vi "Send Callback Message.vi"(8 "error in (no error)":errorcluster, 11 "Order Item in":refnum<class "Order Item.lvclass">) -> (0 "error out":errorcluster, 3 "Order Item out":refnum<class "Order Item.lvclass">)   [LabVIEW 2023, in "Order Item.lvclass"]
doc: "Send the callback message provided by the caller. This enables a zero-coupling relationship between the caller and the callee."
uses:
  Order Item.lvclass
  Order Item.lvclass/Order Item.ctl
  <vilib>/ActorFramework/Self-Addressed Msg/Self-Addressed Msg.lvclass
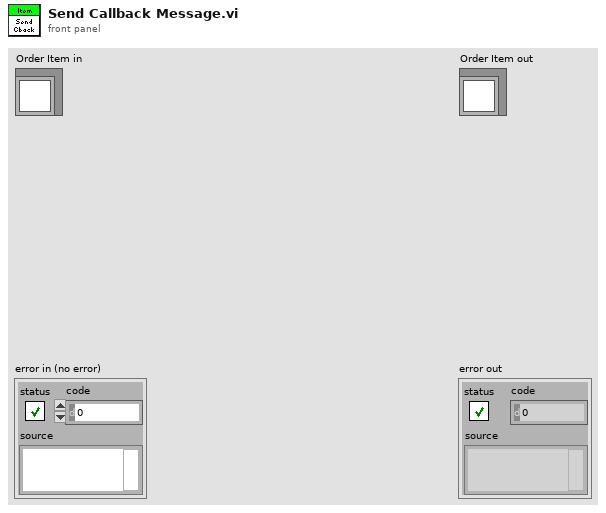
[diagram p1: front panel]
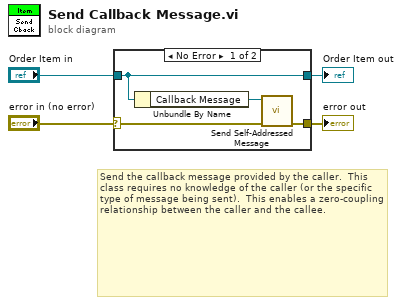
[diagram p0: block diagram]
diagram:
  # "Send the callback message provided by the caller.  This class requires no knowledge of the caller (or the specific type of message being sent).  This enables a zero-coupling relationship between the caller and the callee."
  n1 = case shown="No Error" "error in (no error)" {
    selector: "error in (no error)" -> [w6 w10]
    tunnel: [w5 w10] -> w3
    tunnel: [w8 w9] -> w1
    tunnel: "Order Item in" -> [w8 w9]
    frame No Error {
      n2 = Unbundle By Name(w8) -> ("Callback Message"=w7:refnum<class "Self-Addressed Msg.lvclass">)
      n3 = call-dynamic "Send Self-Addressed Message.vi"("error in (no error)"=w6, "Self-Addressed Message in"=w7) -> ("error out"=w5:errorcluster)  [unwired: 8 in, 1 out]
    }
    frame Error {
    }
  }
  "error out" <- w3
  "Order Item out" <- w1
